vi "AutoDistanceGyro.vi"(0 "InitialAngle":dbl, 1 "Reset Encoders":bool, 2 "Sensor (Gyro)":enum16{"Gyro", "Encoder"}(ring), 5 "TargetDistance":dbl, 7 "Motor Speed":dbl=0.8, 11 "error in":errorcluster) -> (4 "InitialAngle Out":dbl, 15 "error out":errorcluster)   [LabVIEW 2012]
doc: "This VI is called when autonomous begins, and will automatically be terminated when autonomous ends. You can carry out timed or sensor driven robot movement independently without needing to return to the caller."
uses:
  <vilib>/Rock Robotics/WPI/RobotDrive/WPI_RobotDriveGetSetRefNum.vi
  <vilib>/Rock Robotics/WPI/RobotDrive/WPI_RobotDriveArcadeDrive_Standard(NoSaturation).vi
panel:
  in  "PID gains":T1={"proportional gain (Kc)"=0.05000000000000001, "integral time (Ti, min)"=0.006499999999999995, "derivative time (Td, min)"=0.001} {"proportional gain (Kc)" format="%_6g"; "integral time (Ti, min)" format="%_6g"; "derivative time (Td, min)" format="%_6g"}
  out "Distance (ft)":dbl
  out "OutputGraph":T2(graph)
  out "Current Angle":dbl
  out "Current Distance":dbl
  out "Angle Delta":dbl
  out "PID Output":dbl format="%.2f"
  # "Inputs"
  # "Outputs"
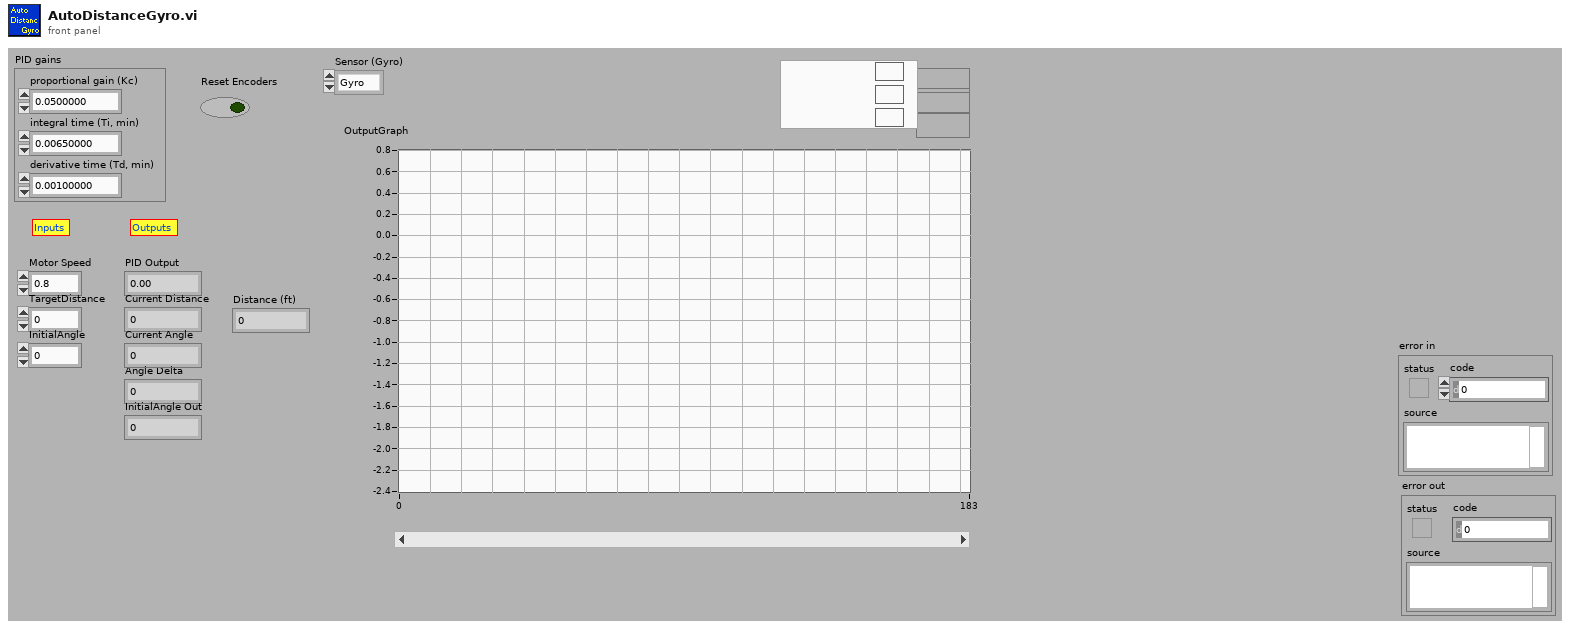
[diagram p1: front panel]
types:
  T1 = cluster{"proportional gain (Kc)":dbl, "integral time (Ti, min)":dbl, "derivative time (Td, min)":dbl}
  T2 = cluster{"Angle":dbl, "InitialAngle":dbl, "output":dbl}
  T3 = typedef "WPI_RobotDriveDevRef.ctl" = cluster{"DevStatus":errorcluster, "Motors[]":T4[], "Square Inputs":bool, "Max Output":dbl, "Isochronous":bool}
  T4 = typedef "WPI_MotorControlDeviceRef.ctl" = cluster{"DeviceStatus":errorcluster, "Type":enum16{"PWM", "CAN"}, "PWM":cluster{"Digital Module":T5, "PWM Channel":T6, "DeadBand":T7}, "CAN":cluster{"Device Number":u8, "Control Mode":T8, "Semaphore":T9, "Max Vout":dbl}, "Invert":bool, "TransformRef":T10, "InvTransformRef":T10}
  T5 = typedef "FPGA_TypedefDigitalModule.ctl" = enum16{"Digital Module 1", "Digital Module 2"}
  T6 = typedef "FPGA_DIOPWMChannel.ctl" = enum8{"PWM 1", "PWM 2", "PWM 3", "PWM 4", "PWM 5", "PWM 6", "PWM 7", "PWM 8", "PWM 9", "PWM 10", "Invalid"}
  T7 = typedef "WPI_PWMDeadband.ctl" = cluster{"Name":string, "maxPositivePwm":i32, "minPositivePwm":i32, "centerPwm":i32, "maxNegativePwm":i32, "minNegativePwm":i32, "angularRange":u16}
  T8 = typedef "WPI_CANJaguar_ControlMode.ctl" = enum8{"Percent VBus", "Current", "Speed", "Position", "Voltage"}
  T9 = typedef "Semaphore RefNum" = refnum<k1>
  T10 = typedef "WPI_PWMTransform_ConPane.ctl" = refnum<vi>
  T11 = typedef "WPI_GyroDevRef.ctl" = cluster{"DevStatus":errorcluster, "Analog Module":T12, "Analog Channel":T13, "Offset":dbl, "Gain (VoltsPerDegree/Second)":dbl}
  T12 = typedef "FPGA_TypedefAnalogModule.ctl" = enum16{"Analog Module 1", "Analog Module 2"}
  T13 = typedef "FPGA_AIChannel.ctl" = enum8{"AI 1", "AI 2", "AI 3", "AI 4", "AI 5", "AI 6", "AI 7", "AI 8", "Invalid"}
  T14 = cluster{"Output":dbl, "InitialAngle":dbl, "Output":dbl}
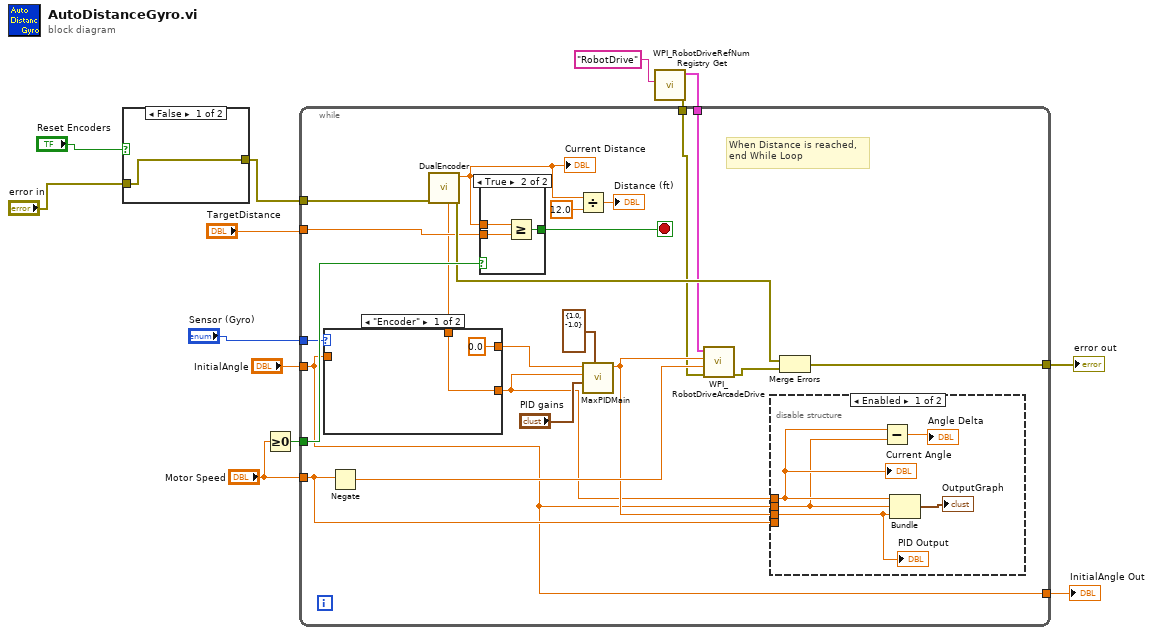
[diagram p0: block diagram]
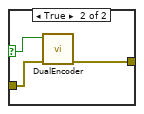
[diagram p2: hidden frame]
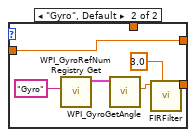
[diagram p3: hidden frame]
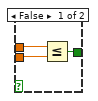
[diagram p4: hidden frame]
diagram:
  n1 = case shown="False" "Reset Encoders" {
    selector: "Reset Encoders" -> [_ w15]
    tunnel: "error in" -> [w14 w17]
    tunnel: [w14 w16] -> w4
    frame False {
    }
    frame True {
      n2 = call "DualEncoder.vi"("error in (no error)"=w17, "Reset?"=w15) -> ("error out"=w16:errorcluster)  [unwired: 5 in, 4 out]
    }
  }
  n3 = Greater Or Equal To 0?(x="Motor Speed") -> (x >= 0?=w10:bool)
  n4 = call <vilib>:"WPI_RobotDriveRefNum Registry Get.vi"("refnum name"="RobotDrive") -> ("error out"=w7:errorcluster, "RobotDriveDevRef"=w8:T3)  [unwired: 9 in]
  n5 = while {
    tunnel: "Motor Speed" -> [w36]
    tunnel: "TargetDistance" -> [w22]
    tunnel: "InitialAngle" -> [w19]
    tunnel: [w19] -> w11
    tunnel: w10 -> [w31]
    tunnel: [w27] -> w9
    tunnel: w4 -> [w28]
    tunnel: w8 -> [w26]
    tunnel: w7 -> [w24]
    tunnel: "Sensor (Gyro)" -> [w21]
    stop <- w39 stop-if-true
    # "When Distance is reached, end While Loop"
    n6 = Negate(x=w36) -> (-x=w37:dbl)
    n7 = call "DualEncoder.vi"("error in (no error)"=w28) -> ("error out"=w29:errorcluster, "Total Distance (in)"=w25:dbl, "Angle (degrees)"=w20:dbl)  [unwired: 6 in, 2 out]
    "Current Distance" <- w25
    n8 = case shown="\"Encoder\"" w21 {
      tunnel: [w41 w44] -> w23
      tunnel: w20 -> [w41 _]
      tunnel: w19 -> [_ w42]
      tunnel: [0.0 ("InitialAngle") w42] -> w18
      frame "Encoder" {
      }
      frame "Gyro", Default {
        n9 = call <vilib>:"WPI_GyroRefNum Registry Get.vi"("refnum name"="Gyro") -> ("GyroDevRef"=w46:T11)  [unwired: 9 in, 1 out]
        n10 = call <vilib>:"WPI_GyroGetAngle.vi"("GyroDevRef"=w46) -> ("Angle"=w45:dbl)  [unwired: 1 in, 9 out]
        n11 = call "FIRFilter.vi"("Filter Size"=3.0, "Input"=w45) -> ("Output"=w44:dbl)  [unwired: 9 in]
      }
    }
    n12 = case shown="True" w31 {
      tunnel: [w50 w53] -> w39
      tunnel: w25 -> [w49 w52]
      tunnel: w22 -> [w48 w51]
      frame False {
        n13 = Less Or Equal?(x=w49, y=w48) -> (x <= y?=w50:bool)
      }
      frame True {
        n14 = Greater Or Equal?(x=w52, y=w51) -> (x >= y?=w53:bool)
      }
    }
    n15 = Divide(x=w25, y=12.0) -> (x/y=→"Distance (ft)":dbl)
    n16 = call "MaxPIDMain.vi"("Output Range"=cluster{"output high":dbl, "output low":dbl} {"output high"=1.0, "output low"=-1.0} ("output range"), "PID gains"="PID gains", "process variable"=w23, "setpoint"=w18) -> ("Output"=w34:dbl)  [unwired: 6 in, 1 out]
    n17 = call-poly <vilib>:"WPI_RobotDriveArcadeDrive.vi"("error in (no error)"=w24, "Y axis value"=w37, "X axis value"=w34, "RobotDriveDevRef"=w26) -> ("error out"=w30:errorcluster)  [unwired: 5 in, 2 out]
    n18 = disable-structure shown="Enabled" {
      disable-tunnel: w23 -> [w55 _]
      disable-tunnel: w19 -> [w54 _]
      disable-tunnel: w36 -> [_ _]
      disable-tunnel: w34 -> [w57 _]
      frame Enabled {
        n19 = Subtract(x=w55, y=w54) -> (x-y=→"Angle Delta":dbl)
        n20 = Bundle("Output"=w55, "InitialAngle"=w54, "Output"=w57) -> (→"OutputGraph":T14)  [unwired: 1 out]
        "PID Output" <- w57
        "Current Angle" <- w55
      }
      frame Disabled {
      }
    }
    n21 = Merge Errors(w29, w30) -> (w27:errorcluster)
  }
  "error out" <- w9
  "InitialAngle Out" <- w11
